vi "Initialize Routing and Faulting Engine.vi"(8 "error in (no error)":errorcluster, 9 "Device Inputs FIFO":refnum<k33>, 10 "Device Outputs FIFO":refnum<k33>, 11 "Device Ref in":T13 format="%.0x") -> (0 "error out":errorcluster, 2 "Engine Data":T1, 3 "Device Ref out":T13 format="%.0x")   [LabVIEW 2020, in "Routing and Faulting Engine.lvlib"]
uses:
  Routing and Faulting Engine.lvlib
  <vilib>/NI VeriStand/Custom Device API/Custom Device Item Ref.ctl
  Engine Data.ctl
  Includes/CDMessaging.lvlibp/Producer/Abstract Producer/Abstract Producer.lvclass
  Shared/Compiled.Settings.ctl
  Shared/Communication Configuration.ctl
  Shared/Routing and Faulting Configuration.ctl
  Shared/Routing Channel Configuration.ctl
  Shared/Value-Connections Map.ctl
  Shared/Alias Mapping.ctl
  Shared/Alias Endpoint.ctl
  Shared/Compiled Connection.ctl
  Shared/FIFO Indices.ctl
  Device Inputs.ctl
  Device Outputs.ctl
  Device FIFOs.ctl
  Shared/Constants.vi
  <vilib>/NI VeriStand/Custom Device API/Get Item Property (Variant).vi
  Shared/Routing and Faulting Shared.lvlib
  <vilib>/NI VeriStand/Custom Device API/Custom Device API.lvlib
  Includes/CDMessaging.lvlibp/Message/Abstract Message/Abstract Message.lvclass
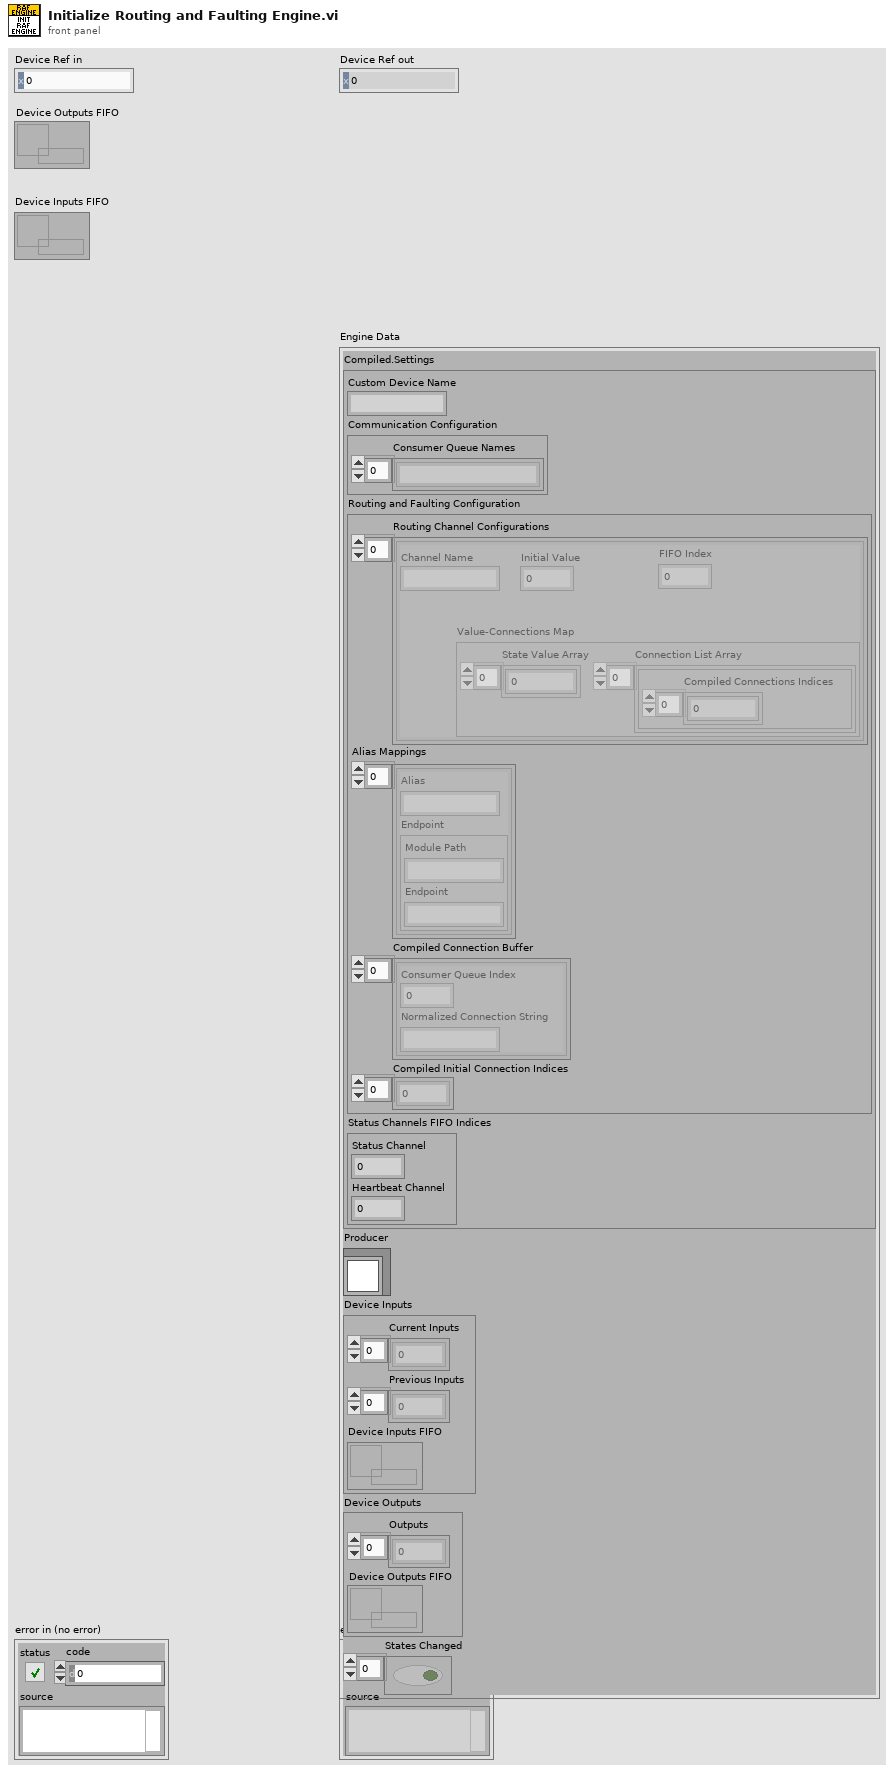
[diagram p1: front panel]
types:
  T1 = typedef "Routing and Faulting Engine.lvlib/Engine Data.ctl" = cluster{"Compiled.Settings":T2, "Producer":refnum<class "Abstract Producer.lvclass">, "Device Inputs":T11, "Device Outputs":T12, "States Changed":bool[]}
  T2 = typedef "Routing and Faulting Shared.lvlib/Compiled.Settings.ctl" = cluster{"Custom Device Name":string, "Communication Configuration":T3, "Routing and Faulting Configuration":T4, "Status Channels FIFO Indices":T10}
  T3 = typedef "Routing and Faulting Shared.lvlib/Communication Configuration.ctl" = cluster{"Consumer Queue Names":string[]}
  T4 = typedef "Routing and Faulting Shared.lvlib/Routing and Faulting Configuration.ctl" = cluster{"Routing Channel Configurations":T5[], "Alias Mappings":T7[], "Compiled Connection Buffer":T9[], "Compiled Initial Connection Indices":i32[]}
  T5 = typedef "Routing and Faulting Shared.lvlib/Routing Channel Configuration.ctl" = cluster{"Channel Name":string, "Initial Value":dbl, "FIFO Index":i32, "Value-Connections Map":T6}
  T6 = typedef "Routing and Faulting Shared.lvlib/Value-Connections Map.ctl" = cluster{"State Value Array":i32[], "Connection List Array":cluster{"Compiled Connections Indices":i32[]}[]}
  T7 = typedef "Routing and Faulting Shared.lvlib/Alias Mapping.ctl" = cluster{"Alias":string, "Endpoint":T8}
  T8 = typedef "Routing and Faulting Shared.lvlib/Alias Endpoint.ctl" = cluster{"Module Path":string, "Endpoint":string}
  T9 = typedef "Routing and Faulting Shared.lvlib/Compiled Connection.ctl" = cluster{"Consumer Queue Index":i32, "Normalized Connection String":string}
  T10 = typedef "Routing and Faulting Shared.lvlib/FIFO Indices.ctl" = cluster{"Status Channel":i32, "Heartbeat Channel":i32}
  T11 = typedef "Routing and Faulting Engine.lvlib/Device Inputs.ctl" = cluster{"Current Inputs":dbl[], "Previous Inputs":dbl[], "Device Inputs FIFO":refnum<k33>}
  T12 = typedef "Routing and Faulting Engine.lvlib/Device Outputs.ctl" = cluster{"Outputs":dbl[], "Device Outputs FIFO":refnum<k33>}
  T13 = typedef "Custom Device API.lvlib/Custom Device Item Ref.ctl" = u64
  T14 = typedef "Routing and Faulting Engine.lvlib/Device FIFOs.ctl" = cluster{"Device Inputs FIFO":refnum<k33>, "Device Outputs FIFO":refnum<k33>}
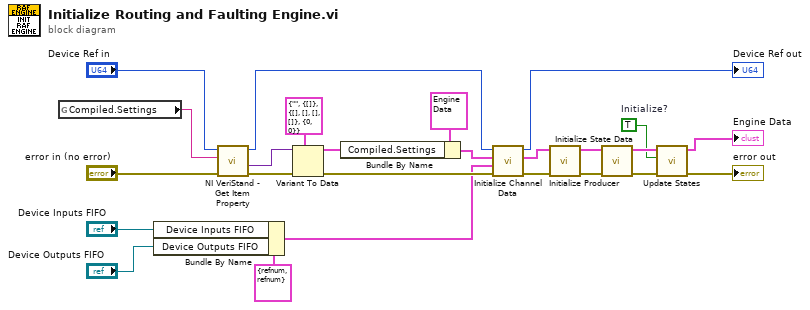
[diagram p0: block diagram]
diagram:
  w1 = TRUE  # Initialize?
  n1 = global read "Constants.vi" "Compiled.Settings"() -> (w25:string)
  n2 = Bundle By Name(cluster=T14 {"Device Inputs FIFO"=refnum, "Device Outputs FIFO"=refnum} ("Device FIFOs"), "Device Inputs FIFO"="Device Inputs FIFO", "Device Outputs FIFO"="Device Outputs FIFO") -> (w9:T14)
  n3 = call-poly <vilib>:"NI VeriStand - Get Item Property.vi"("error in (no error)"="error in (no error)", "Property Name"=w25, "Item Ref in"="Device Ref in") -> ("error out"=w23:errorcluster, "Value"=w22:variant, "Item Ref out"=w15:T13)  [unwired: 5 in, 1 out]
  n4 = Variant To Data(error in=w23, type=T2 {"Custom Device Name"="", "Communication Configuration"={"Consumer Queue Names"=[]}, "Routing and Faulting Configuration"={"Routing Channel Configurations"=[], "Alias Mappings"=[], "Compiled Connection Buffer"=[], "Compiled Initial Connection Indices"=[]}, "Status Channels FIFO Indices"={"Status Channel"=0, "Heartbeat Channel"=0}} ("Compiled.Settings"), Variant=w22) -> (data=w18:T2, error out=w20:errorcluster)
  n5 = Bundle By Name(cluster=T1 {"Compiled.Settings"={"Custom Device Name"="", "Communication Configuration"={"Consumer Queue Names"=[]}, "Routing and Faulting Configuration"={"Routing Channel Configurations"=[], "Alias Mappings"=[], "Compiled Connection Buffer"=[], "Compiled Initial Connection Indices"=[]}, "Status Channels FIFO Indices"={"Status Channel"=0, "Heartbeat Channel"=0}}, "Producer"=refnum, "Device Inputs"={"Current Inputs"=[], "Previous Inputs"=[], "Device Inputs FIFO"=refnum}, "Device Outputs"={"Outputs"=[], "Device Outputs FIFO"=refnum}, "States Changed"=[]} ("Engine Data"), "Compiled.Settings"=w18) -> (w17:T1)
  n6 = call "Initialize Channel Data.vi"("error in (no error)"=w20, "FIFOs"=w9, "Engine Data in"=w17, "Device Ref in"=w15) -> ("error out"=w13:errorcluster, "Engine Data out"=w7:T1, "Device Ref out"=→"Device Ref out":T13)  [unwired: 5 in]
  n7 = call "Initialize Producer.vi"("error in (no error)"=w13, "Engine Data in"=w7) -> ("error out"=w8:errorcluster, "Engine Data out"=w6:T1)  [unwired: 8 in]
  n8 = call "Initialize State Data.vi"("error in (no error)"=w8, "Engine Data in"=w6) -> ("error out"=w5:errorcluster, "Engine Data out"=w3:T1)  [unwired: 8 in]
  n9 = call "Update States.vi"("error in (no error)"=w5, "Initialize?"=w1, "Engine Data in"=w3) -> ("error out"=→"error out":errorcluster, "Engine Data out"=→"Engine Data":T1)  [unwired: 7 in]
